vi "PlayerJoinTest.vi"() -> ()   [LabVIEW 2025]
uses:
  common/CommonClientNetworkInterfaceGlobalVariables.vi
panel:
  out "Sent Message":string
  out "Return message":string
  in  "Player name":string
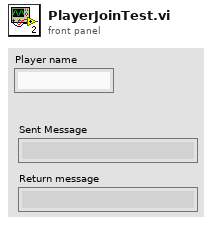
[diagram p1: front panel]
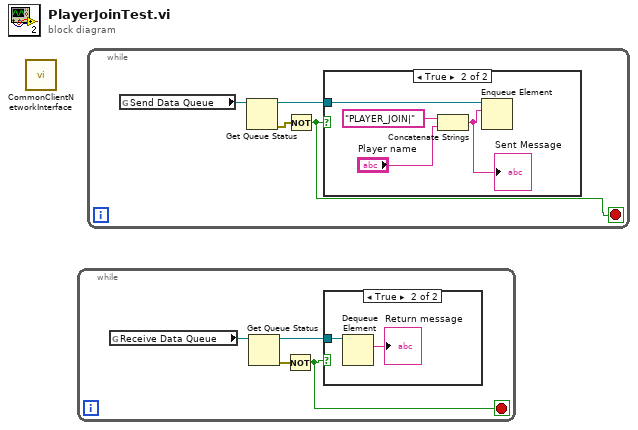
[diagram p0: block diagram]
diagram:
  n1 = call "CommonClientNetworkInterface.vi"() -> ()  [unwired: 1 in]
  n2 = while {
    stop <- w1 stop-if-true
    n3 = global read "CommonClientNetworkInterfaceGlobalVariables.vi" "Receive Data Queue"() -> (w4:refnum<queue>)
    n4 = Get Queue Status(queue=w4) -> (queue out=w3:refnum<queue>, error out=w2:errorcluster)  [unwired: 2 in, 6 out]
    n5 = Not(x=w2) -> (.not. x?=w1:bool)
    n6 = case shown="True" w1 {
      tunnel: w3 -> [_ w5]
      frame False {
      }
      frame True {
        n7 = Dequeue Element(queue=w5) -> (element=→"Return message":string)  [unwired: 2 in, 3 out]
      }
    }
  }
  n8 = while {
    stop <- w7 stop-if-true
    n9 = global read "CommonClientNetworkInterfaceGlobalVariables.vi" "Send Data Queue"() -> (w10:refnum<queue>)
    n10 = Get Queue Status(queue=w10) -> (queue out=w9:refnum<queue>, error out=w8:errorcluster)  [unwired: 2 in, 6 out]
    n11 = Not(x=w8) -> (.not. x?=w7:bool)
    n12 = case shown="True" w7 {
      tunnel: w9 -> [_ w12]
      frame False {
      }
      frame True {
        n13 = Concatenate Strings("PLAYER_JOIN|" ("string"), "Player name") -> (w11:string)
        "Sent Message" <- w11
        n14 = Enqueue Element(queue=w12, element=w11) -> ()  [unwired: 2 in, 3 out]
      }
    }
  }
